vi "niRFUtil RFHS Fine Tune Resampler.vi"(0 "Complex Waveform In":T1={"x0"=0.0, "dx"=1.0, "y"=[]} {"y" format="%.2f"; "dx" format="%^.2e"; "x0" format="%^.2e"}, 2 "CPU Context":string="M1 1", 5 "Sample Rate Error (ppm)":dbl format="%#_6p", 7 "Initial Sample Offset (samples)":dbl format="%#_6p", 11 "error in (no error)":errorcluster, 12 "Allowable Sampling Rate Error (ppm)":dbl=1.0 format="%_2g") -> (4 "Complex Waveform Out":T1 {"y" format="%.2f"; "dx" format="%^.2e"; "x0" format="%^.2e"}, 15 "error out":errorcluster)   [LabVIEW 2015, in "niRFUtil.lvlib"]
doc: "Wrapper for quickly using the niRFHS Channelizer as resampler."
uses:
  niRFUtil.lvlib
  Includes/niRFUtil INC Complex Waveform.ctl
  Includes/niRFUtil INC Complex Array.ctl
  Includes/niRFUtil RFHS Channelizer FilterTypeHint.ctl
  Includes/niRFUtil RFHS Channelizer ChannelSpecification.ctl
  Includes/niRFUtil RFHS Channelizer ChannelSpecificationBase.ctl
  Includes/niRFUtil RFHS Channelizer ChannelFlags.ctl
  Includes/niRFUtil RFHS Channelizer ChannelizerBufferingMode.ctl
  Includes/niRFUtil RFHS Channelizer FilterPurpose.ctl
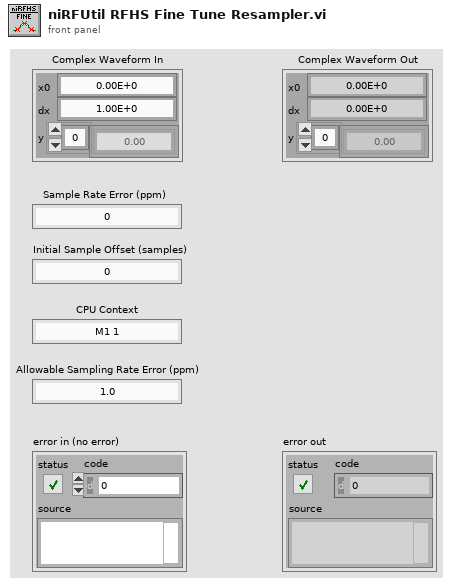
[diagram p1: front panel]
types:
  T1 = typedef "niRFUtil.lvlib/niRFUtil INC Complex Waveform.ctl" = cluster{"x0":dbl, "dx":dbl, "y":T2}
  T2 = typedef "niRFUtil.lvlib/niRFUtil INC Complex Array.ctl" = csg[]
  T3 = typedef "niRFUtil.lvlib/niRFUtil RFHS Channelizer FilterPurpose.ctl" = enum16{"Channelizer", "Fine Tune Resampler"}
  T4 = typedef "niRFUtil.lvlib/niRFUtil RFHS Channelizer ChannelizerBufferingMode.ctl" = enum32{"Unbuffered", "Finite", "Continuous"}
  T5 = typedef "niRFUtil.lvlib/niRFUtil RFHS Channelizer ChannelSpecification.ctl" = cluster{"freq in Hz":bool, "Filter Type Hint":T6, "Hint Value":dbl, "Channels":T7[]}
  T6 = typedef "niRFUtil.lvlib/niRFUtil RFHS Channelizer FilterTypeHint.ctl" = enum16{"Auto", "FFT (LTE)", "FFT (WiFi)", "FFT (custom)"}
  T7 = typedef "niRFUtil.lvlib/niRFUtil RFHS Channelizer ChannelSpecificationBase.ctl" = cluster{"fc":dbl, "fs":dbl, "passBW":dbl, "stopBW":dbl, "Rejection (dB)":dbl, "Flags":T8, "Reserved":i32}
  T8 = typedef "niRFUtil.lvlib/niRFUtil RFHS Channelizer ChannelFlags.ctl" = u32
  T9 = typedef "niRFUtil.lvlib/niRFUtil RFHS Filter Pre Post Trigger Info.ctl" = cluster{"Pre-trigger Len (input)":i64, "Min Post-trigger Len (input)":i64}
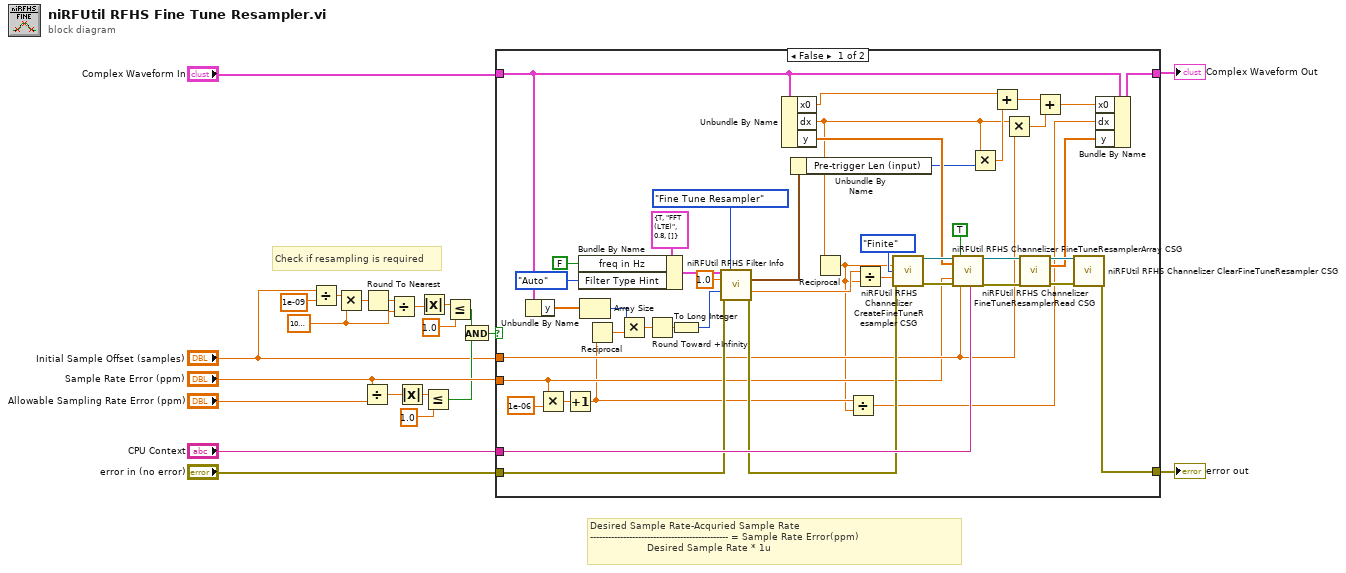
[diagram p0: block diagram]
diagram:
  w11 = 1000000.0 ("y")
  # "Desired Sample Rate-Acquried Sample Rate\n---------------------------------------------- = Sample Rate Error(ppm)\n                   Desired Sample Rate * 1u"
  # "Check if resampling is required"
  n1 = Divide(x="Initial Sample Offset (samples)", y=1e-09 ("upper limit")) -> (x/y=w6:dbl)
  n2 = Multiply(x=w6, y=w11) -> (x*y=w9:dbl)
  n3 = Divide(x="Sample Rate Error (ppm)", y="Allowable Sampling Rate Error (ppm)") -> (x/y=w3:dbl)
  n4 = Round To Nearest(number=w9) -> (nearest integer value=w10:dbl)
  n5 = Divide(x=w10, y=w11) -> (x/y=w12:dbl)
  n6 = Absolute Value(x=w3) -> (abs(x)=w14:dbl)
  n7 = Absolute Value(x=w12) -> (abs(x)=w7:dbl)
  n8 = Less Or Equal?(x=w14, y=1.0) -> (x <= y?=w15:bool)
  n9 = Less Or Equal?(x=w7, y=1.0) -> (x <= y?=w5:bool)
  n10 = And(x=w5, y=w15) -> (x .and. y?=w2:bool)
  n11 = case shown="False" w2 {
    tunnel: [w67 w69] -> w22
    tunnel: "Complex Waveform In" -> [w41 w69]
    tunnel: "CPU Context" -> [w66 _]
    tunnel: [w65 w68] -> w20
    tunnel: "error in (no error)" -> [w64 w68]
    tunnel: "Initial Sample Offset (samples)" -> [w36 _]
    tunnel: "Sample Rate Error (ppm)" -> [w32 _]
    frame False {
      n12 = Unbundle By Name(w41) -> ("y"=w40:T2)
      n13 = Multiply(x=w32, y=1e-06 ("x")) -> (x*y=w34:dbl)
      n14 = Increment(x=w34) -> (x+1=w26:dbl)
      n15 = Bundle By Name(cluster=T5 {"freq in Hz"=TRUE, "Filter Type Hint"=enum."FFT (LTE)", "Hint Value"=0.8, "Channels"=[]} ("Channel Spec"), "freq in Hz"=FALSE, "Filter Type Hint"=niRFUtil_RFHS_Channelizer_FilterTypeHint."Auto") -> (w42:T5)
      n16 = Array Size(array=w40) -> (size(s)=w28:i32)
      n17 = Reciprocal(x=w26) -> (1/x=w29:dbl)
      n18 = Multiply(x=w28, y=w29) -> (x*y=w31:dbl)
      n19 = Round Toward +Infinity(x=w31) -> (ceil(x): smallest int >= x=w30:dbl)
      n20 = To Long Integer(number=w30) -> (32bit integer=w27:i32)
      n21 = call "niRFUtil RFHS Filter Info.vi"("Channelizer Spec"=w42, "Filter Purpose"=niRFUtil_RFHS_Channelizer_FilterPurpose."Fine Tune Resampler", "fs [Hz]"=1.0, "#output samples"=w27, "error in (no error)"=w64) -> ("Pre/Post Trigger Filter Info"=w48:T9, "#input samples (#output samples)"=w47:dbl, "error out"=w50:errorcluster)  [unwired: 6 in, 2 out]
      n22 = Unbundle By Name(w41) -> ("x0"=w44:dbl, "dx"=w25:dbl, "y"=w49:T2)
      n23 = Unbundle By Name(w48) -> ("Pre-trigger Len (input)"=w45:i64)
      n24 = Reciprocal(x=w25) -> (1/x=w23:dbl)
      n25 = Divide(x=w26, y=w23) -> (x/y=w24:dbl)
      n26 = Divide(x=w47, y=w23) -> (x/y=w58:dbl)
      n27 = call "niRFUtil RFHS Channelizer CreateFineTuneResampler CSG.vi"("fs [Hz]"=w23, "Mode"=niRFUtil_RFHS_Channelizer_ChannelizerBufferingMode."Finite", "Buffer Size (s)"=w58, "error in (no error)"=w50) -> ("Resampler Ref"=w59:refnum<data-value>, "error out"=w52:errorcluster)  [unwired: 10 in]
      n28 = call "niRFUtil RFHS Channelizer FineTuneResamplerArray CSG.vi"("Resampler Ref"=w59, "Data"=w49, "fs shift (ppm)"=w32, "error in (no error)"=w52, "Reset"=TRUE, "phase shift (samples)"=w36, "CPU Context"=w66) -> ("Resampler Ref (out)"=w55:refnum<data-value>, "error out"=w54:errorcluster)  [unwired: 9 in, 2 out]
      n29 = Multiply(x=w25, y=w45) -> (x*y=w43:dbl)
      n30 = Add(x=w44, y=w43) -> (x+y=w38:dbl)
      n31 = Multiply(x=w25, y=w36) -> (x*y=w35:dbl)
      n32 = call "niRFUtil RFHS Channelizer FineTuneResamplerRead CSG.vi"("Resampler Ref"=w55, "error in (no error)"=w54) -> ("Resampler Ref (out)"=w57:refnum<data-value>, "Channel Data"=w53:csg[], "error out"=w56:errorcluster)  [unwired: 11 in]
      n33 = Add(x=w38, y=w35) -> (x+y=w37:dbl)
      n34 = call "niRFUtil RFHS Channelizer ClearFineTuneResampler CSG.vi"("Resampler Ref"=w57, "error in (no error)"=w56) -> ("error out"=w65:errorcluster)  [unwired: 12 in, 1 out]
      n35 = Bundle By Name(cluster=w41, "x0"=w37, "dx"=w24, "y"=w53) -> (w67:T1)
    }
    frame True {
    }
  }
  "error out" <- w20
  "Complex Waveform Out" <- w22
